vi "CONF chanel config routing.vi"(7 "Route array":i32[](array[numeric])=[1, 3, 5, 7, 8, 6, 4, 2], 8 "error in (no error)":errorcluster, 10 "AI HW conf array in":T1[](array[typedef])) -> (0 "error out":errorcluster, 2 "AI HW conf array out":T1[](array[typedef]))   [LabVIEW 2013]
doc: "zmienia kolejnoœæ kana³ów do konfiguracji\nDomyœlna kolejnoœæ kana³ów: 1, 3, 5, 7, 8, 6, 4, 2"
uses:
  Kontrolki/KartaDAQ/CONF AI HW config.ctl
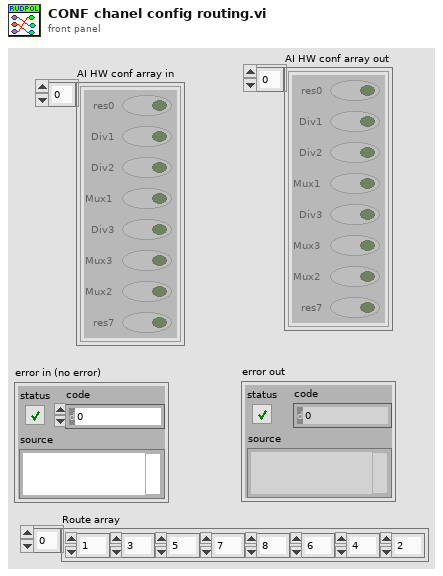
[diagram p1: front panel]
types:
  T1 = typedef "CONF AI HW config.ctl" = cluster{"res0":bool, "Div1":bool, "Div2":bool, "Mux1":bool, "Div3":bool, "Mux3":bool, "Mux2":bool, "res7":bool}
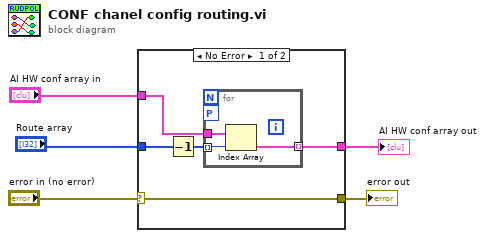
[diagram p0: block diagram]
diagram:
  n1 = case shown="No Error" "error in (no error)" {
    selector: "error in (no error)" -> [w6 w14]
    tunnel: [w10 w15] -> w2
    tunnel: "Route array" -> [w9 _]
    tunnel: "AI HW conf array in" -> [w7 w15]
    tunnel: [w6 w14] -> w3
    frame No Error {
      n2 = Decrement(x=w9) -> (x-1=w8:i32[])
      n3 = for {
        tunnel: w8 -> [w13] mode=indexing
        tunnel: w7 -> [w12]
        tunnel: [w11] -> w10 mode=indexing
        workers-P: _ -> [_]
        n4 = Index Array(array=w12, index=w13) -> (element=w11:T1)
      }
    }
    frame Error {
    }
  }
  "error out" <- w3
  "AI HW conf array out" <- w2
